vi "read camera settingssub.vi"(0 "camera session  in":T1, 1 "error in":errorcluster) -> (2 "camera session out":T1, 3 "error out":errorcluster, 4 "Camera settings":T2={"Pixel format"=1, "exposure time [microsec]"=20.0, "Exposure time setting"=1, "gain [dB]"=0.0, "Auto Gain"=1, "Gamma enable"=FALSE, "gamma "=0.25, "ISP enable "=FALSE, "black level clamping enabled"=FALSE, "black level (%)"=0.0, "binning vertical"=1, "binning hor"=1, "vertical binning mode"=1, "horizontal  binning mode"=1, "width"=8.0, "height "=4.0, "max width"=8.0, "max height"=8.0, "exposure time vis"=enum."Enabled", "gain vis"=enum."Enabled", "vert binning vis"=[], "hor bin  vis"=[], "gamma vis"=enum."Enabled", "black level vis"=enum."Enabled"} {"max height" min=0.0 max=1330.0; "max width" min=0.0 max=1150.0; "height" min=0.0 max=1330.0; "horizontal  binning mode" items=["Additive", "Average"]; "vertical binning mode" items=["Additive", "Average"]; "binning hor" items=["1", "2", "4"]; "binning vertical" items=["1", "2", "4"]; "black level (%)" min=-5.0 max=10.0; "gamma" min=0.25 max=4.0 step=0.1; "Auto Gain" items=["Continuous", "Once", "Off"]; "gain [dB]" min=0.0 max=47.0; "Exposure time setting" items=["Continuous", "Once", "Off"]; "exposure time [microsec]" min=20.0 max=30000000.0; "Pixel format" items=["Mono8", "Mono16", "Mono10Packed", "Mono12Packed", "Mono10p", "Mono12p"]})   [LabVIEW 2018]
uses:
  read settings control.ctl
  <vilib>/userdefined/High Color/IMAQdx.ctl
  <resource>/objmgr/imaqdx.rc
  <vilib>/vision/driver/NI_Vision_Acquisition_Software.lvlib
panel:
  out "index of element":i32
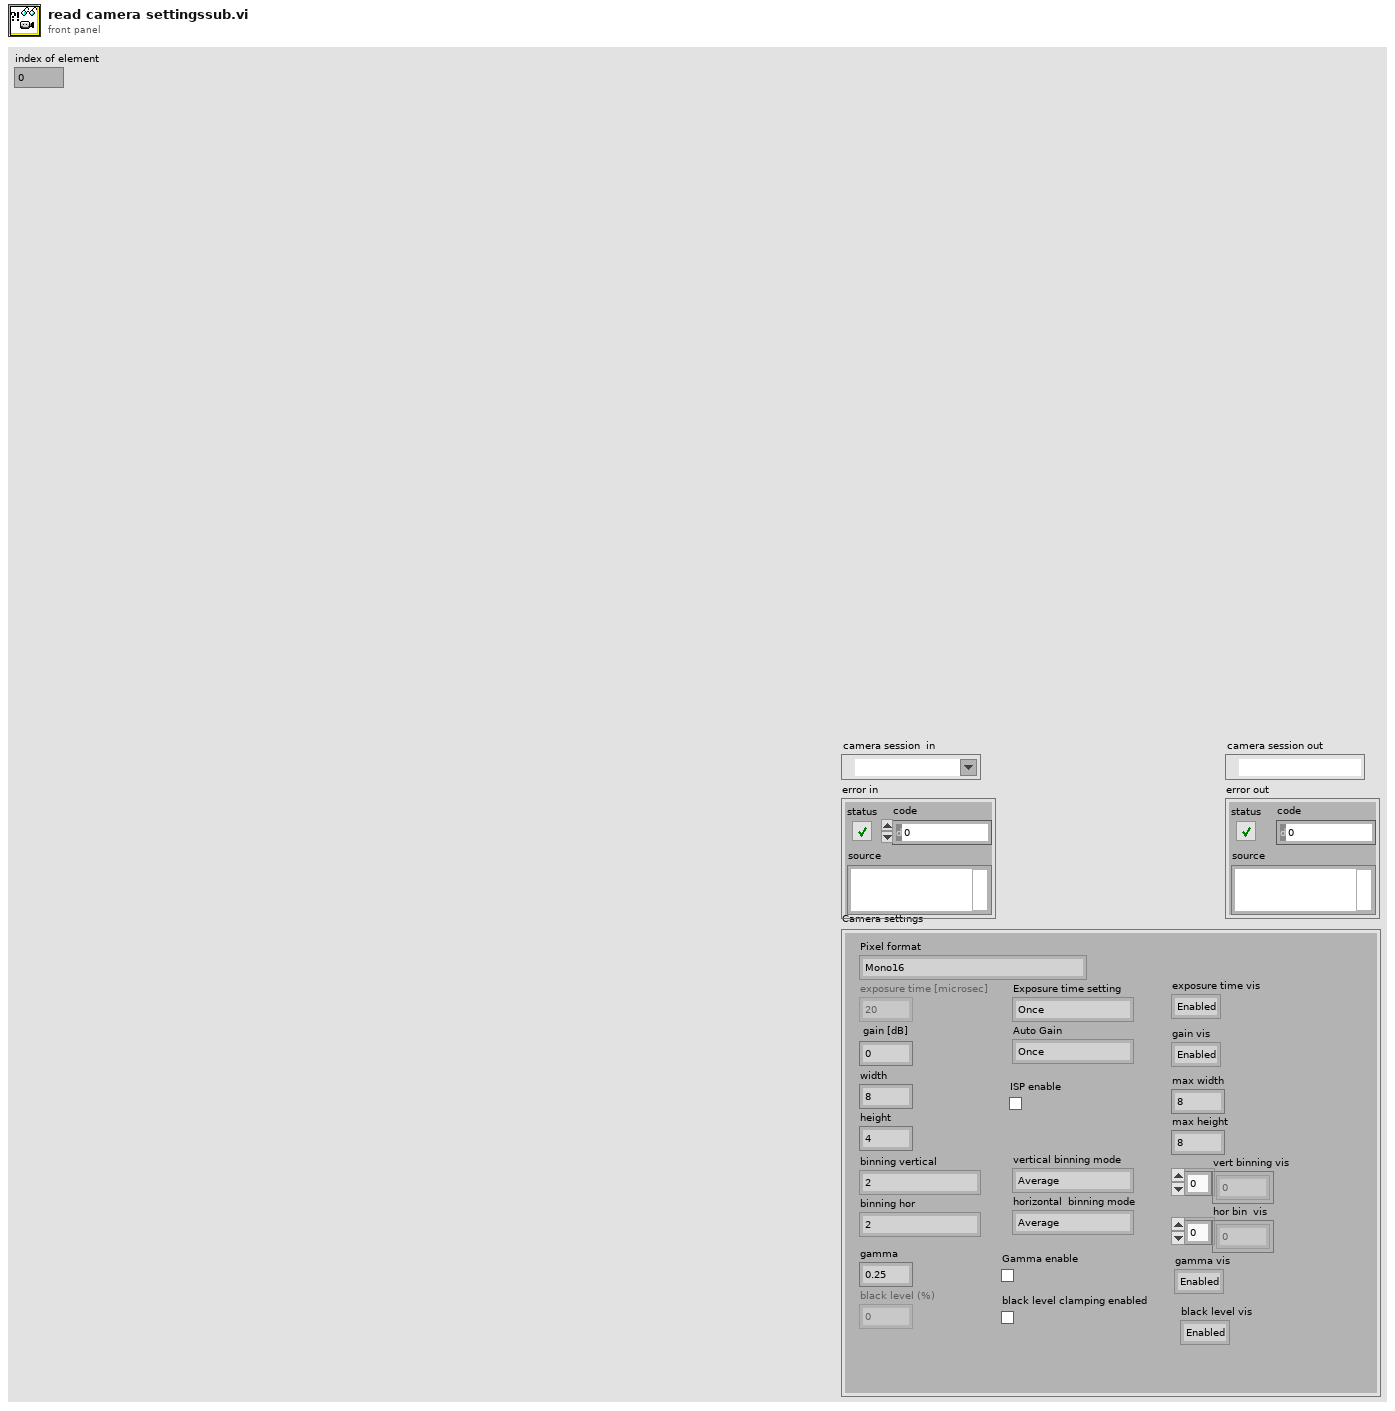
[diagram p1: front panel]
types:
  T1 = typedef "IMAQdx.ctl" = refnum<k21>
  T2 = typedef "read settings control.ctl" = cluster{"Pixel format":u16, "exposure time [microsec]":dbl, "Exposure time setting":u16, "gain [dB]":dbl, "Auto Gain":u16, "Gamma enable":bool, "gamma ":dbl, "ISP enable ":bool, "black level clamping enabled":bool, "black level (%)":dbl, "binning vertical":u16, "binning hor":u16, "vertical binning mode":u16, "horizontal  binning mode":u16, "width":dbl, "height ":dbl, "max width":dbl, "max height":dbl, "exposure time vis":enum8{"Enabled", "Disabled", "Disabled and Grayed Out"}, "gain vis":enum8{"Enabled", "Disabled", "Disabled and Grayed Out"}, "vert binning vis":i32[], "hor bin  vis":i32[], "gamma vis":enum8{"Enabled", "Disabled", "Disabled and Grayed Out"}, "black level vis":enum8{"Enabled", "Disabled", "Disabled and Grayed Out"}}
  T3 = enum8{"Enabled", "Disabled", "Disabled and Grayed Out"}
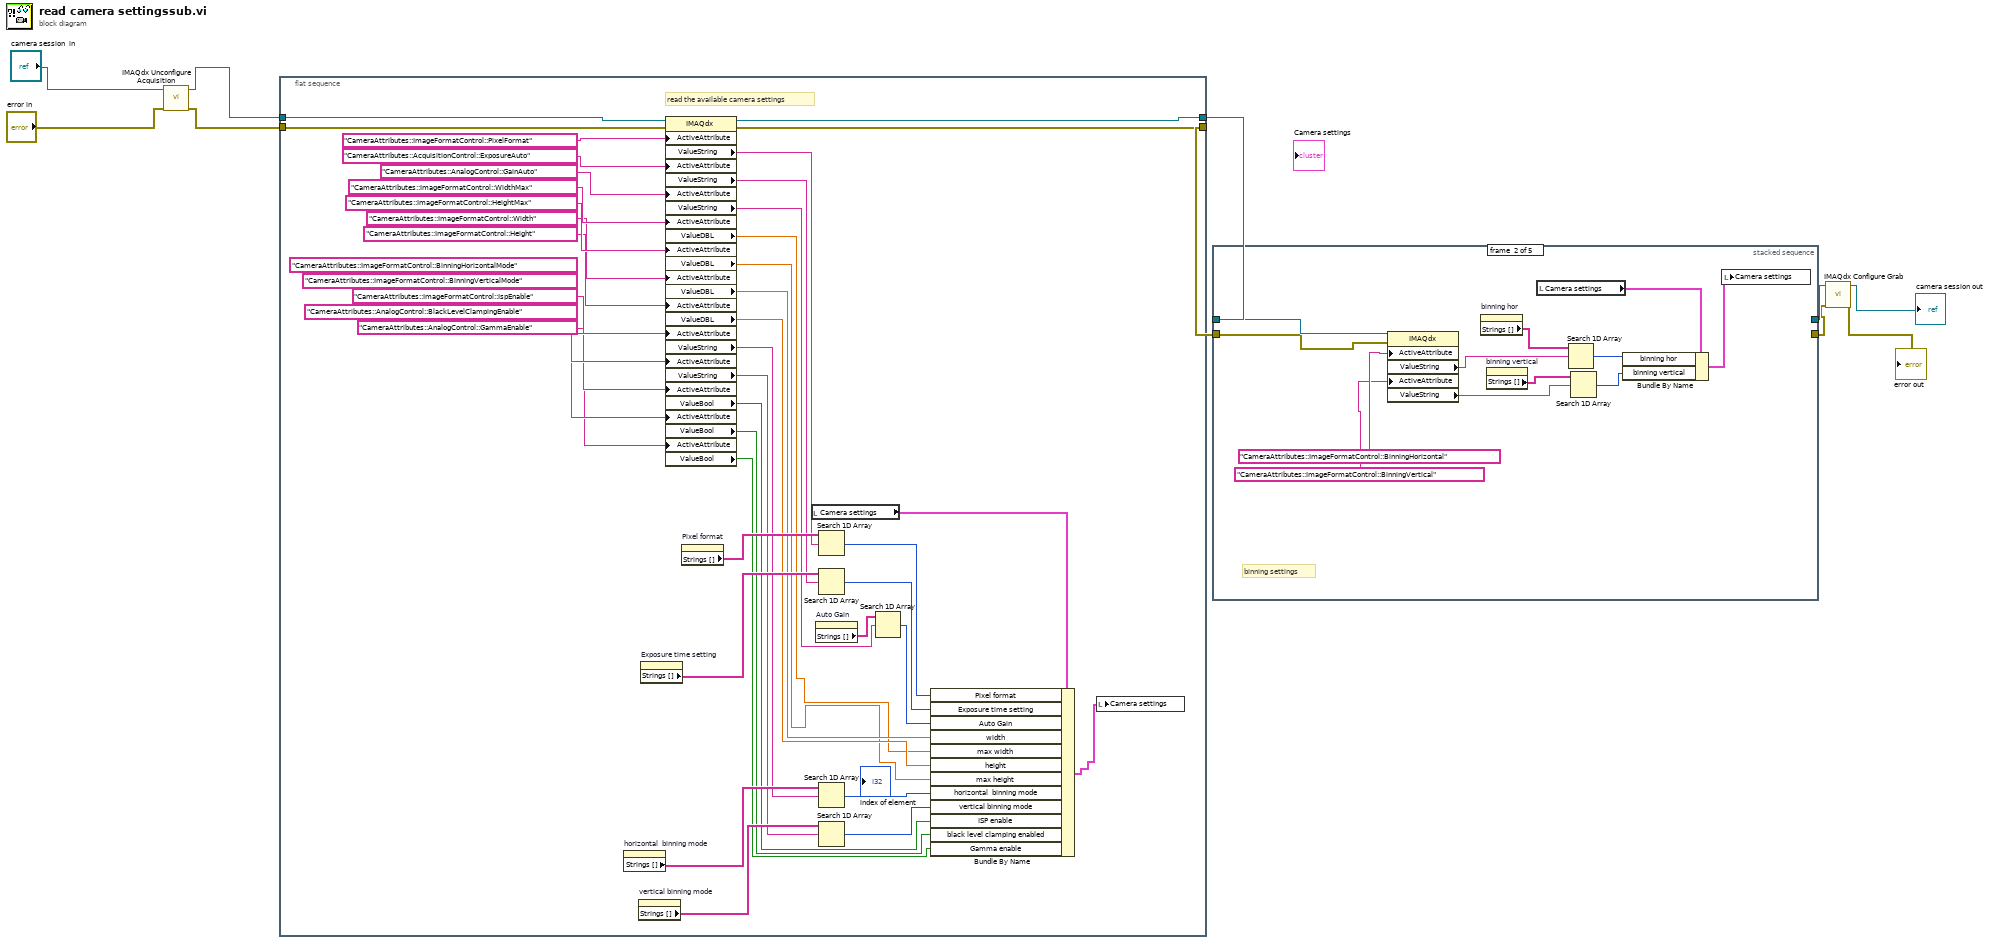
[diagram p0: block diagram]
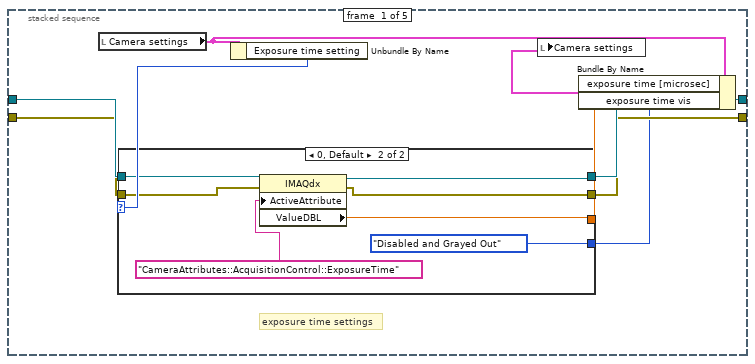
[diagram p2: hidden frame]
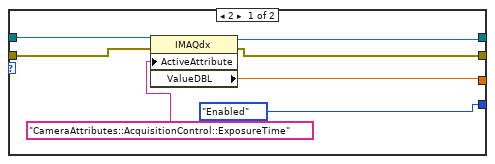
[diagram p3: hidden frame]
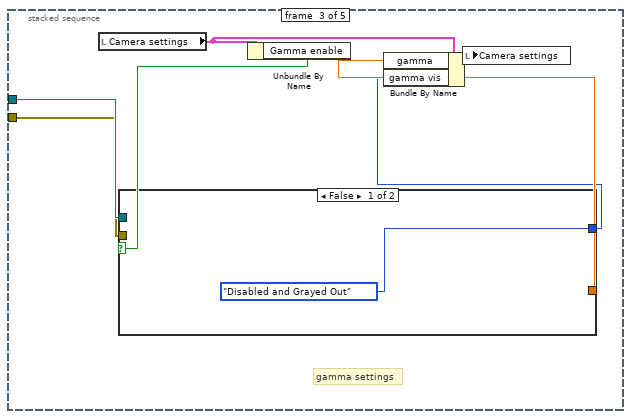
[diagram p4: hidden frame]
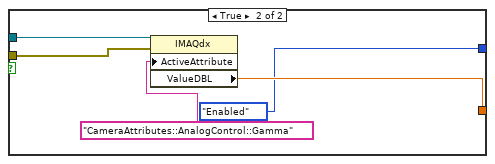
[diagram p5: hidden frame]
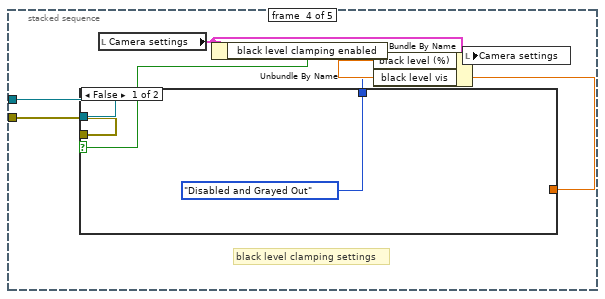
[diagram p6: hidden frame]
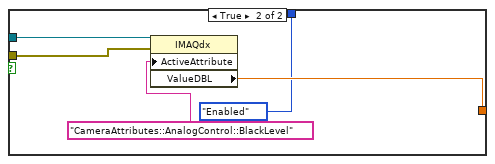
[diagram p7: hidden frame]
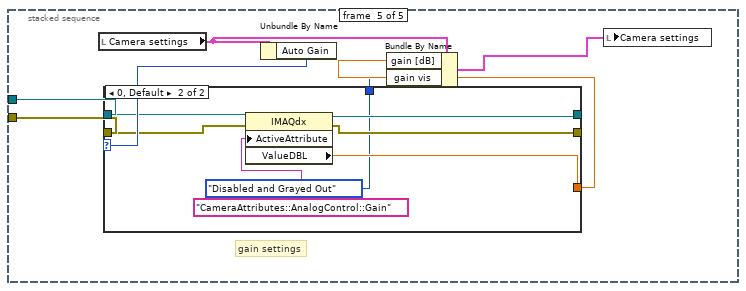
[diagram p8: hidden frame]
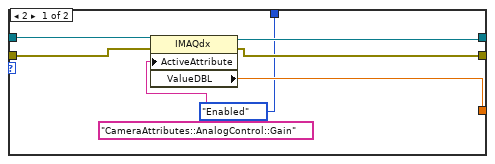
[diagram p9: hidden frame]
diagram:
  n1 = call <vilib>:"IMAQdx Unconfigure Acquisition.vi"("error in"="error in", "Session In"="camera session  in") -> ("error out"=w7:errorcluster, "Session Out"=w8:T1)  [unwired: 8 in]
  n2 = flat-sequence {
    tunnel: w8 -> [w50]
    tunnel: w7 -> [w49]
    tunnel: [w18] -> w10
    tunnel: [w17] -> w9
    frame #0 {
      # "read the available camera settings"
      n3 = property on="horizontal  binning mode" class="Ring (strict)"() -> ("Strings []"=w30:string[])  [unwired: 2 in, 2 out]
      n4 = property on="vertical binning mode" class="Ring (strict)"() -> ("Strings []"=w27:string[])  [unwired: 2 in, 2 out]
      n5 = property on="Exposure time setting" class="Ring (strict)"() -> ("Strings []"=w43:string[])  [unwired: 2 in, 2 out]
      n6 = property class="IMAQdx"(reference=w50, error in=w49, "ActiveAttribute"="CameraAttributes::ImageFormatControl::PixelFormat", "ActiveAttribute"="CameraAttributes::AcquisitionControl::ExposureAuto", "ActiveAttribute"="CameraAttributes::AnalogControl::GainAuto", "ActiveAttribute"="CameraAttributes::ImageFormatControl::WidthMax", "ActiveAttribute"="CameraAttributes::ImageFormatControl::HeightMax", "ActiveAttribute"="CameraAttributes::ImageFormatControl::Width", "ActiveAttribute"="CameraAttributes::ImageFormatControl::Height", "ActiveAttribute"="CameraAttributes::ImageFormatControl::BinningHorizontalMode", "ActiveAttribute"="CameraAttributes::ImageFormatControl::BinningVerticalMode", "ActiveAttribute"="CameraAttributes::ImageFormatControl::IspEnable", "ActiveAttribute"="CameraAttributes::AnalogControl::BlackLevelClampingEnable", "ActiveAttribute"="CameraAttributes::AnalogControl::GammaEnable") -> (reference out=w18:T1, error out=w17:errorcluster, "ValueString"=w46:string, "ValueString"=w42:string, "ValueString"=w39:string, "ValueDBL"=w13:dbl, "ValueDBL"=w12:dbl, "ValueDBL"=w34:dbl, "ValueDBL"=w33:dbl, "ValueString"=w29:string, "ValueString"=w26:string, "ValueBool"=w23:bool, "ValueBool"=w20:bool, "ValueBool"=w19:bool)
      n7 = property on="Pixel format" class="Ring (strict)"() -> ("Strings []"=w47:string[])  [unwired: 2 in, 2 out]
      n8 = local read "Camera settings"() -> (w16:T2)
      n9 = property on="Auto Gain" class="Ring (strict)"() -> ("Strings []"=w40:string[])  [unwired: 2 in, 2 out]
      n10 = Search 1D Array(1D array=w47, element=w46) -> (index of element=w45:i32)  [unwired: 1 in]
      n11 = Search 1D Array(1D array=w43, element=w42) -> (index of element=w14:i32)  [unwired: 1 in]
      n12 = Search 1D Array(1D array=w30, element=w29) -> (index of element=w28:i32)  [unwired: 1 in]
      n13 = Search 1D Array(1D array=w27, element=w26) -> (index of element=w25:i32)  [unwired: 1 in]
      n14 = Search 1D Array(1D array=w40, element=w39) -> (index of element=w15:i32)  [unwired: 1 in]
      n15 = Bundle By Name(cluster=w16, "Pixel format"=w45, "Exposure time setting"=w14, "Auto Gain"=w15, "width"=w34, "max width"=w13, "height"=w33, "max height"=w12, "horizontal  binning mode"=w28, "vertical binning mode"=w25, "ISP enable"=w23, "black level clamping enabled"=w20, "Gamma enable"=w19) -> (w11:T2)
      n16 = local write "Camera settings"(w11) -> ()
    }
  }
  n17 = stacked-sequence {
    tunnel: w10 -> [w58 w85 w91 w104 w117]
    tunnel: w9 -> [w57 w84 w90 w103 w116]
    tunnel: [w56 _ _ _ _] -> w6
    tunnel: [w55 _ _ _ _] -> w5
    frame #0 {
      # "exposure time settings"
      n18 = local read "Camera settings"() -> (w53:T2)
      n19 = Unbundle By Name(w53) -> ("Exposure time setting"=w59:u16)
      n20 = case shown="0, Default" w59 {
        tunnel: w58 -> [w66 w73]
        tunnel: w57 -> [w65 w72]
        tunnel: [w64 w71] -> w56
        tunnel: [w63 w70] -> w55
        tunnel: [w61 w68] -> w52
        tunnel: [T3."Enabled" ("Disabled") T3."Disabled and Grayed Out" ("Disabled")] -> w51
        frame 2 {
          n21 = property class="IMAQdx"(reference=w66, error in=w65, "ActiveAttribute"="CameraAttributes::AcquisitionControl::ExposureTime") -> (reference out=w64:T1, error out=w63:errorcluster, "ValueDBL"=w61:dbl)
        }
        frame 0, Default {
          n22 = property class="IMAQdx"(reference=w73, error in=w72, "ActiveAttribute"="CameraAttributes::AcquisitionControl::ExposureTime") -> (reference out=w71:T1, error out=w70:errorcluster, "ValueDBL"=w68:dbl)
        }
      }
      n23 = Bundle By Name(cluster=w53, "exposure time [microsec]"=w52, "exposure time vis"=w51) -> (w54:T2)
      n24 = local write "Camera settings"(w54) -> ()
    }
    frame #1 {
      # "binning settings"
      n25 = property class="IMAQdx"(reference=w85, error in=w84, "ActiveAttribute"="CameraAttributes::ImageFormatControl::BinningHorizontal", "ActiveAttribute"="CameraAttributes::ImageFormatControl::BinningVertical") -> ("ValueString"=w81:string, "ValueString"=w79:string)  [unwired: 2 out]
      n26 = property on="binning hor" class="Ring (strict)"() -> ("Strings []"=w80:string[])  [unwired: 2 in, 2 out]
      n27 = property on="binning vertical" class="Ring (strict)"() -> ("Strings []"=w78:string[])  [unwired: 2 in, 2 out]
      n28 = local read "Camera settings"() -> (w74:T2)
      n29 = Search 1D Array(1D array=w80, element=w81) -> (index of element=w76:i32)  [unwired: 1 in]
      n30 = Search 1D Array(1D array=w78, element=w79) -> (index of element=w75:i32)  [unwired: 1 in]
      n31 = Bundle By Name(cluster=w74, "binning hor"=w76, "binning vertical"=w75) -> (w77:T2)
      n32 = local write "Camera settings"(w77) -> ()
    }
    frame #2 {
      # "gamma settings"
      n33 = local read "Camera settings"() -> (w88:T2)
      n34 = Unbundle By Name(w88) -> ("Gamma enable"=w92:bool)
      n35 = case shown="False" w92 {
        tunnel: w91 -> [_ w98]
        tunnel: w90 -> [_ w97]
        tunnel: [_ w95] -> w87
        tunnel: [T3."Disabled and Grayed Out" ("Disabled") T3."Enabled" ("Disabled")] -> w86
        frame False {
        }
        frame True {
          n36 = property class="IMAQdx"(reference=w98, error in=w97, "ActiveAttribute"="CameraAttributes::AnalogControl::Gamma") -> ("ValueDBL"=w95:dbl)  [unwired: 2 out]
        }
      }
      n37 = Bundle By Name(cluster=w88, "gamma"=w87, "gamma vis"=w86) -> (w89:T2)
      n38 = local write "Camera settings"(w89) -> ()
    }
    frame #3 {
      # "black level clamping settings"
      n39 = local read "Camera settings"() -> (w101:T2)
      n40 = Unbundle By Name(w101) -> ("black level clamping enabled"=w105:bool)
      n41 = case shown="False" w105 {
        tunnel: w104 -> [_ w111]
        tunnel: w103 -> [_ w110]
        tunnel: [_ w108] -> w100
        tunnel: [T3."Disabled and Grayed Out" ("Disabled") T3."Enabled" ("Disabled")] -> w99
        frame False {
        }
        frame True {
          n42 = property class="IMAQdx"(reference=w111, error in=w110, "ActiveAttribute"="CameraAttributes::AnalogControl::BlackLevel") -> ("ValueDBL"=w108:dbl)  [unwired: 2 out]
        }
      }
      n43 = Bundle By Name(cluster=w101, "black level (%)"=w100, "black level vis"=w99) -> (w102:T2)
      n44 = local write "Camera settings"(w102) -> ()
    }
    frame #4 {
      # "gain settings"
      n45 = local read "Camera settings"() -> (w114:T2)
      n46 = Unbundle By Name(w114) -> ("Auto Gain"=w118:u16)
      n47 = case shown="0, Default" w118 {
        tunnel: w117 -> [w125 w132]
        tunnel: w116 -> [w124 w131]
        tunnel: [w123 w130] -> _
        tunnel: [w122 w129] -> _
        tunnel: [w120 w127] -> w115
        tunnel: [T3."Enabled" ("Disabled") T3."Disabled and Grayed Out" ("Disabled")] -> w112
        frame 2 {
          n48 = property class="IMAQdx"(reference=w125, error in=w124, "ActiveAttribute"="CameraAttributes::AnalogControl::Gain") -> (reference out=w123:T1, error out=w122:errorcluster, "ValueDBL"=w120:dbl)
        }
        frame 0, Default {
          n49 = property class="IMAQdx"(reference=w132, error in=w131, "ActiveAttribute"="CameraAttributes::AnalogControl::Gain") -> (reference out=w130:T1, error out=w129:errorcluster, "ValueDBL"=w127:dbl)
        }
      }
      n50 = Bundle By Name(cluster=w114, "gain [dB]"=w115, "gain vis"=w112) -> (w113:T2)
      n51 = local write "Camera settings"(w113) -> ()
    }
  }
  n52 = call <vilib>:"IMAQdx Configure Grab.vi"("error in"=w5, "Session In"=w6) -> ("error out"=→"error out":errorcluster, "Session Out"=→"camera session out":T1)  [unwired: 8 in]
